vi "Write Number of Steps.vi"(8 "error in (no error)":errorcluster, 10 "Number of Steps":i32, 11 "Number of Steps in":refnum<class "Number of Steps.lvclass">) -> (0 "error out":errorcluster, 3 "Number of Steps out":refnum<class "Number of Steps.lvclass">)   [LabVIEW 2019, in "TestEngine.lvlib" / "Number of Steps.lvclass"]
uses:
  Number of Steps.lvclass
  Number of Steps.lvclass/Number of Steps.ctl
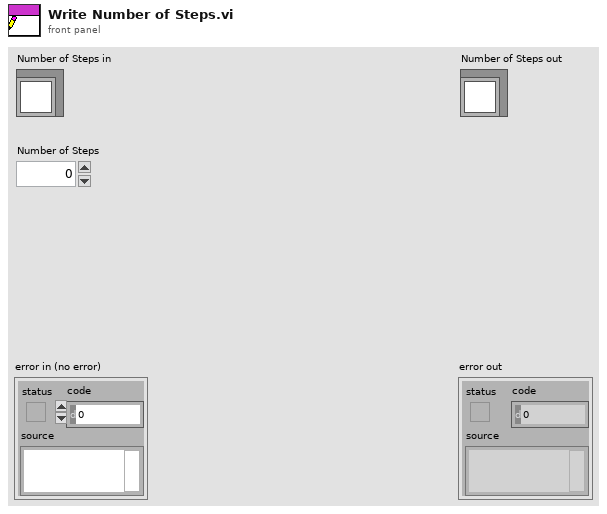
[diagram p1: front panel]
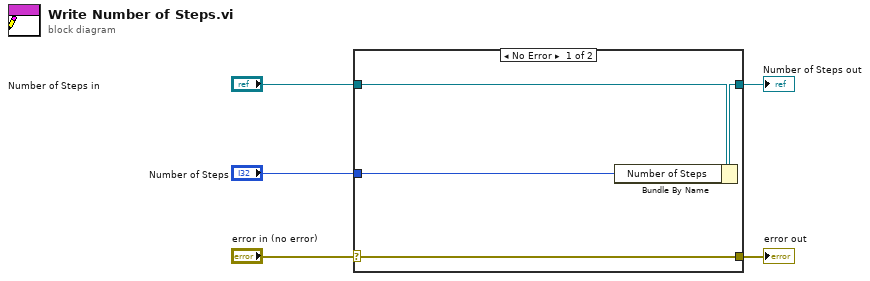
[diagram p0: block diagram]
diagram:
  n1 = case shown="No Error" "error in (no error)" {
    selector: "error in (no error)" -> [w9 w10]
    tunnel: [w9 w10] -> w4
    tunnel: [w7 w11] -> w2
    tunnel: "Number of Steps in" -> [w8 w11]
    tunnel: "Number of Steps" -> [w6 _]
    frame No Error {
      n2 = Bundle By Name(cluster=w8, "Number of Steps"=w6) -> (w7:refnum<class "Number of Steps.lvclass">)
    }
    frame Error {
    }
  }
  "error out" <- w4
  "Number of Steps out" <- w2
